vi "displayErrorMessage.vi"(10 "viewThisComponent":refnum<class "ViewThisComponent.lvclass">) -> ()   [LabVIEW 2016, in "EXAViewElements.lvlib"]
doc: "Displays error messages."
uses:
  EXAViewElements.lvlib
  ViewThisComponent/ViewThisComponent.lvclass
  C:/ApeironSW/CMP_UserEvents/ComponentTemplateCore/ComponentModel/ComponentModel/View/View.lvclass
  ComponentTemplateCore/ComponentModel/ComponentModel/Typedefs/ComponentStateValues.ctl
  <vilib>/Utility/error.llb/DialogType.ctl
  ComponentTemplateCore/ComponentModel/ComponentModel/View/View.lvclass
panel:
  out "ErrorMessage":string caption="Error Message"
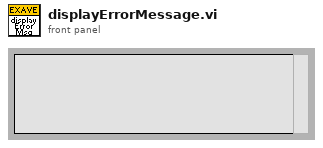
[diagram p1: front panel]
types:
  T1 = typedef "EXATypedefs.lvlib/PubDataEvents.ctl" = cluster{"DetailedState":refnum<user-event>, "ErrorCode":refnum<user-event>, "Heartbeat":refnum<user-event>, "LoopTime_ms":refnum<user-event>, "LoopTimeOutOfRange":refnum<user-event>, "RejectedCommand":refnum<user-event>, "SummaryState":refnum<user-event>, "Timestamp":refnum<user-event>}
  T2 = typedef "componentStateValues.ctl" = enum16{"Off", "Standby", "Enabled", "Disabled", "Fault"}
  T3 = typedef "ComponentStateValues.ctl" = enum16{"Off", "Standby", "Enabled", "Disabled", "Fault"}
  T4 = typedef "DialogType.ctl" = u16
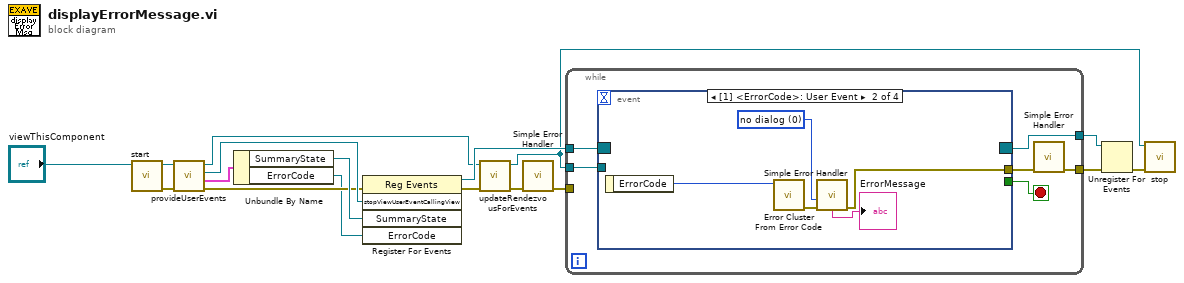
[diagram p0: block diagram]
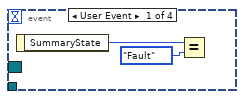
[diagram p2: hidden frame]
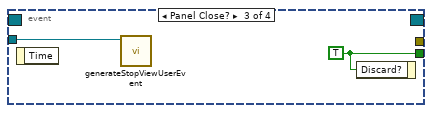
[diagram p3: hidden frame]
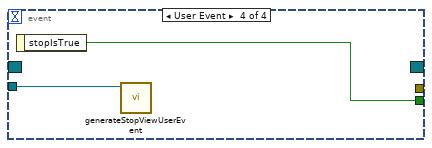
[diagram p4: hidden frame]
diagram:
  n1 = call-dynamic "start.vi"("View in"="viewThisComponent") -> ("error out"=w11:errorcluster, "View out"=w12:refnum<class "ViewThisComponent.lvclass">)  [unwired: 9 in]
  n2 = call "provideUserEvents.vi"("error in (no error)"=w11, "ViewThisComponent in"=w12) -> ("error out"=w13:errorcluster, "pubDataEvents"=w14:T1, "stopViewUserEventCallingView"=w15:refnum<user-event>, "ViewThisComponent out"=w2:refnum<class "ViewThisComponent.lvclass">)  [unwired: 6 in]
  n3 = Unbundle By Name(w14) -> ("SummaryState"=w16:refnum<user-event>, "ErrorCode"=w8:refnum<user-event>)
  n4 = register-events(error in=w13, w15, w16, w8) -> (reference out=w10:refnum<event-registration>, error out=w4:errorcluster)  [unwired: 1 in]
  n5 = call "updateRendezvousForEvents.vi"("error in (no error)"=w4, "View in"=w2) -> ("error out"=w3:errorcluster, "View out"=w1:refnum<class "ViewThisComponent.lvclass">)  [unwired: 8 in]
  n6 = call <vilib>:"Simple Error Handler.vi"("error in (no error)"=w3) -> ("error out"=w7:errorcluster)  [unwired: 4 in, 4 out]
  n7 = while {
    tunnel: w10 -> [w23]
    tunnel: w1 -> [w21]
    tunnel: [w20] -> w5
    tunnel: [w18] -> w9
    tunnel: w7 -> [_]
    stop <- w19 stop-if-true
    n8 = event shown="[1] <ErrorCode>: User Event" {
      selector: w23 -> [_ _ _ _]
      dyn-events: [_ _ _ _] -> w18
      timeout: _ -> [_ _ _ _]
      tunnel: [_ w26 _ _] -> w22
      tunnel: w21 -> [_ _ w32 w33]
      tunnel: [_ _ w31 w34] -> w19
      event User Event {
        n9 = event-data() -> ("SummaryState"=w25:T3)  [unwired: 1 in]
        n10 = Equal?(x=w25, y=componentStateValues."Fault" ("componentStateValues")) -> ()  [unwired: 1 out]
      }
      event User Event {
        w30 = T4 0 items=["no dialog", "OK message", "continue or stop message", "OK message + warnings", "continue/stop + warnings"] ("type of dialog (OK msg:1)")
        n11 = event-data() -> ("ErrorCode"=w27:i32)  [unwired: 1 in]
        n12 = call <vilib>:"Error Cluster From Error Code.vi"("error code (0)"=w27) -> ("error out"=w29:errorcluster)  [unwired: 8 in]
        n13 = call <vilib>:"Simple Error Handler.vi"("type of dialog (OK msg:1)"=w30, "error in (no error)"=w29) -> ("error out"=w26:errorcluster, "message"=→"ErrorMessage":string)  [unwired: 3 in, 3 out]
      }
      event Panel Close? {
        w31 = TRUE ("Discard?")
        n14 = event-data() -> ()  [unwired: 1 in, 1 out]
        n15 = call "generateStopViewUserEvent.vi"("View in"=w32) -> ()  [unwired: 9 in, 2 out]
        n16 = event-data("Discard?"=w31) -> ()  [unwired: 1 in, 1 out]
      }
      event User Event {
        n17 = event-data() -> ("stopIsTrue"=w34:bool)  [unwired: 1 in]
        n18 = call "generateStopViewUserEvent.vi"("View in"=w33) -> ()  [unwired: 9 in, 2 out]
      }
    }
    n19 = call <vilib>:"Simple Error Handler.vi"("error in (no error)"=w22) -> ("error out"=w20:errorcluster)  [unwired: 4 in, 4 out]
  }
  n20 = Unregister For Events(event registration refnum=w9, error in=w5) -> (error out=w6:errorcluster)
  n21 = call-dynamic "stop.vi"("error in (no error)"=w6, "View in"=w1) -> ()  [unwired: 8 in, 2 out]
